vi "Run Transparently.vi"(8 "error in (no error)":errorcluster, 11 "This VI":refnum<vi>) -> (0 "error out":errorcluster={"status"=FALSE, "code"=0, "source"="Property Node (arg 1) in Run Transparently.vi->PC Main.vi\n<APPEND>\nProperty Name: <b>Front Panel Window:Transparency</b>"})   [LabVIEW 2021]
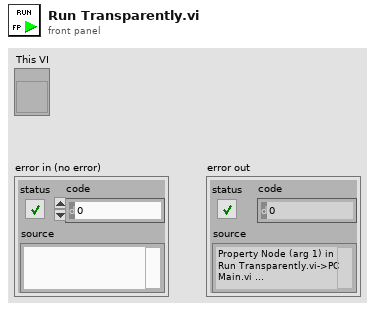
[diagram p1: front panel]
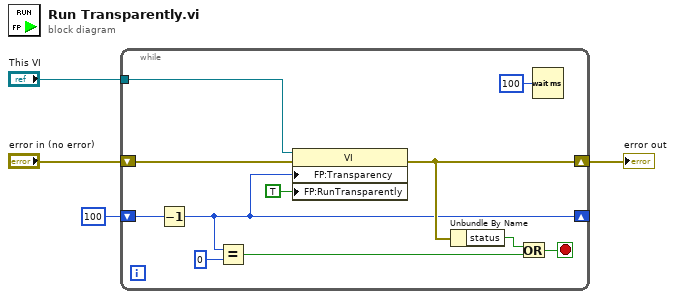
[diagram p0: block diagram]
diagram:
  n1 = while {
    shift-right: [w11] -> w3
    shift-left: "error in (no error)" -> [w5]
    shift-right: [w10] -> _
    shift-left: u8 100 -> [w14]
    tunnel: "This VI" -> [w12]
    stop <- w6 stop-if-true
    n2 = Decrement(x=w14) -> (x-1=w10:u8)
    n3 = Equal?(x=w10, y=u8 0) -> (x = y?=w7:bool)
    n4 = property class="VI"(reference=w12, error in=w5, "FP:Transparency"=w10, "FP:RunTransparently"=TRUE ("Front Panel Window:Run VI Transparently")) -> (error out=w11:errorcluster)  [unwired: 1 out]
    n5 = Unbundle By Name(w11) -> ("status"=w8:bool)
    n6 = Or(x=w8, y=w7) -> (x .or. y?=w6:bool)
    n7 = Wait (ms)(milliseconds to wait=u32 100) -> ()  [unwired: 1 out]
  }
  "error out" <- w3
